vi "Get User Events.vi"(8 "error in (no error)":errorcluster, 11 "User Event in":refnum<class "User Event.lvclass">) -> (0 "error out":errorcluster, 2 "User Events":T1, 3 "User Event out":refnum<class "User Event.lvclass">)   [LabVIEW 2016, in "User Event.lvclass"]
uses:
  User Event.lvclass
  TypeDefs/M1M3SupSimUserEvents.ctl
  TypeDefs/InclinometerResponse.ctl
  TypeDefs/DisplaceResponse.ctl
  TypeDefs/AccelerometerResponse.ctl
  TypeDefs/DigitalInput.ctl
  User Event.lvclass/User Event.ctl
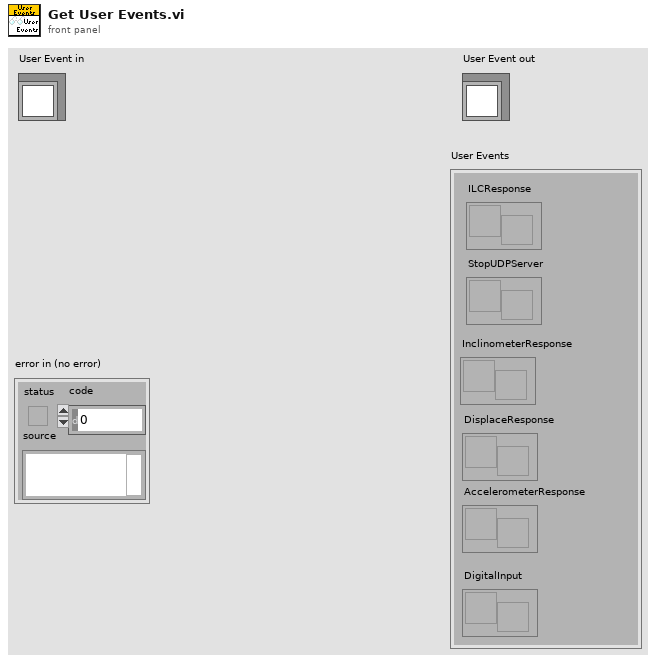
[diagram p1: front panel]
types:
  T1 = typedef "M1M3SupSimUserEvents.ctl" = cluster{"ILCResponse":refnum<user-event>, "StopUDPServer":refnum<user-event>, "InclinometerResponse":refnum<user-event>, "DisplaceResponse":refnum<user-event>, "AccelerometerResponse":refnum<user-event>, "DigitalInput":refnum<user-event>}
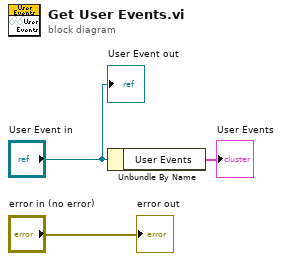
[diagram p0: block diagram]
diagram:
  n1 = Unbundle By Name("User Event in") -> ("User Events"=→"User Events":T1)
  "error out" <- "error in (no error)"
  "User Event out" <- "User Event in"
